vi "invert_bit_14.vi"(11 "Pockels Level(14 bit)":dbl) -> (2 "number":u32, 3 "to hex convert":dbl, 4 "bin_out_invert_14":bool[](array[boolean]), 5 "bin_in":bool[](array[boolean]))   [LabVIEW 2020]
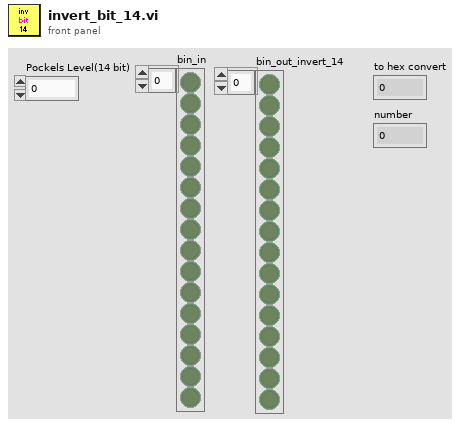
[diagram p1: front panel]
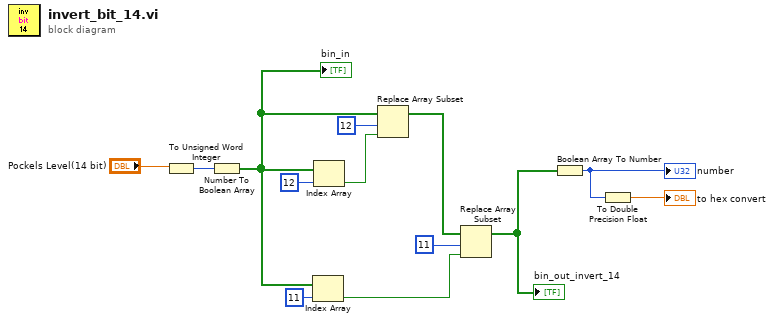
[diagram p0: block diagram]
diagram:
  n1 = To Unsigned Word Integer(number="Pockels Level(14 bit)") -> (unsigned 16bit integer=w12:u16)
  n2 = Number To Boolean Array(number=w12) -> (Boolean array=w9:bool[])
  "bin_in" <- w9
  n3 = Index Array(array=w9, index=11) -> (element=w3:bool)
  n4 = Index Array(array=w9, index=12) -> (element=w1:bool)
  n5 = Replace Array Subset(array=w9, new element=w1, index=12) -> (w5:bool[])
  n6 = Replace Array Subset(array=w5, new element=w3, index=11) -> (w2:bool[])
  "bin_out_invert_14" <- w2
  n7 = Boolean Array To Number(Boolean array=w2) -> (number=w11:u32)
  "number" <- w11
  n8 = To Double Precision Float(number=w11) -> (double precision float=→"to hex convert":dbl)
